vi "Matlab Script.vi"(0 "Xr":dbl[](array[numeric]), 1 "Yr":dbl[](array[numeric]), 2 "Xy":dbl[](array[numeric]), 3 "Yy":dbl[](array[numeric]), 4 "Xw":dbl[](array[numeric]), 5 "Yw":dbl[](array[numeric]), 6 "Couleur Win":u32, 7 "Error In":errorcluster, 10 "Couleur Lose":u32, 11 "Path":path) -> (13 "Error Out":errorcluster, 16 "Script Path 2":path)   [LabVIEW 2025]
doc: "Ce VI construit le script Matlab d’analyse (AnalyseTx.m) à partir des données extraites précédemment\n(Pos.txt) et des paramètres de configuration LabVIEW. Il génère un fichier texte contenant les instructions Matlab prêtes à exécution, en intégrant automatiquement les paramètres. Le fichier Matlab est ensuite enregistré dans le répertoire de travail et sera exécuté par RunMatlab.vi."
panel:
  out "concatenated string":string
  in  "BallminScore":dbl=15.0
  in  "MoveDistPx":dbl=9.0
  in  "BallBorderDist":dbl=9.0
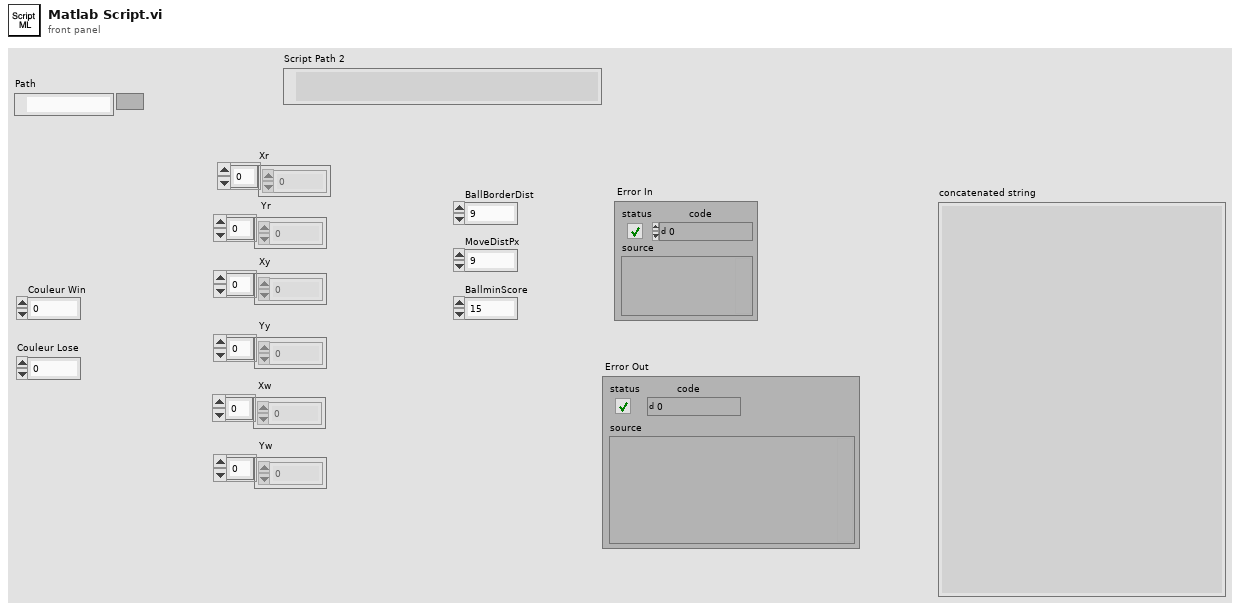
[diagram p1: front panel]
types:
  T1 = enum16{"open", "replace", "create", "open or create", "replace or create", "replace or create with confirmation"}
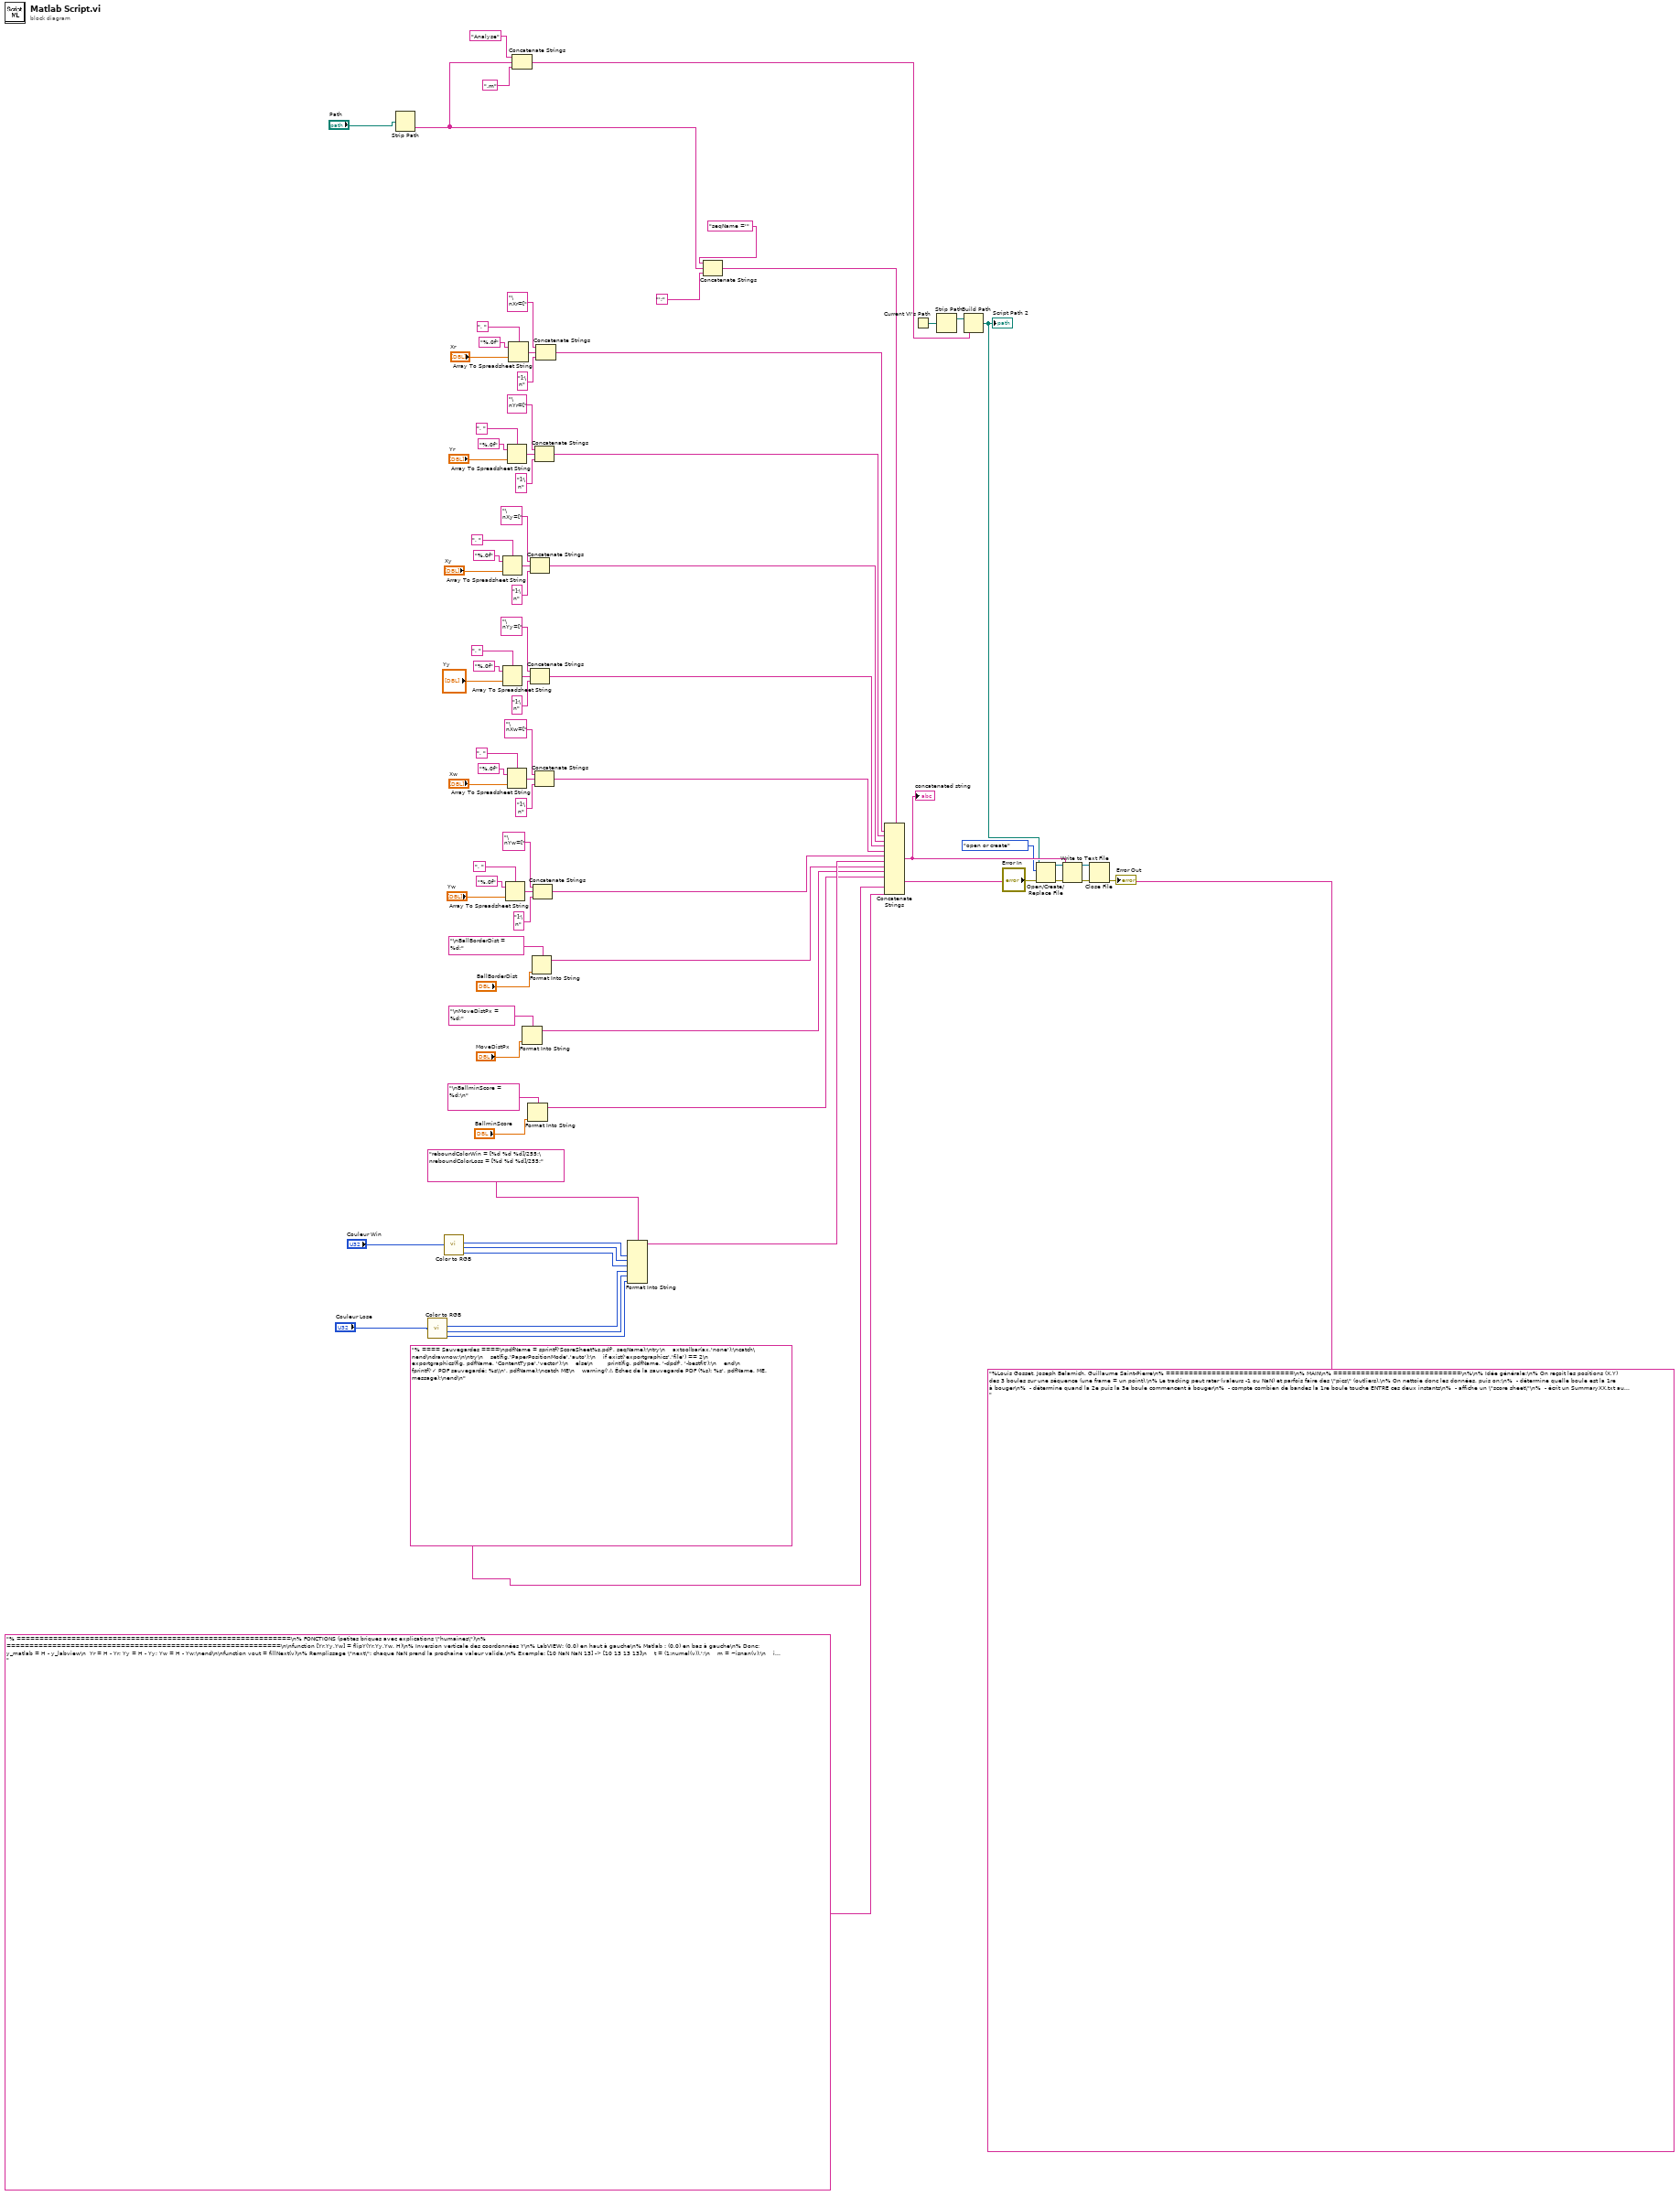
[diagram p0: block diagram]
diagram:
  n1 = Strip Path(path="Path") -> (name=w2:string)  [unwired: 1 out]
  n2 = call <vilib>:"Color to RGB.vi"("Color"="Couleur Lose") -> ("R"=w5:u8, "G"=w4:u8, "B"=w3:u8)  [unwired: 1 out]
  n3 = call <vilib>:"Color to RGB.vi"("Color"="Couleur Win") -> ("R"=w8:u8, "G"=w7:u8, "B"=w6:u8)  [unwired: 1 out]
  n4 = Array To Spreadsheet String(delimiter (Tab)=", ", array="Xy", 3:"%.0f" ("format string")) -> (spreadsheet string=w71:string)
  n5 = Array To Spreadsheet String(delimiter (Tab)=", ", array="Yy", 3:"%.0f" ("format string")) -> (spreadsheet string=w66:string)
  n6 = Array To Spreadsheet String(delimiter (Tab)=", ", array="Yw", 3:"%.0f" ("format string")) -> (spreadsheet string=w56:string)
  n7 = Array To Spreadsheet String(delimiter (Tab)=", ", array="Yr", 3:"%.0f" ("format string")) -> (spreadsheet string=w76:string)
  n8 = Array To Spreadsheet String(delimiter (Tab)=", ", array="Xw", 3:"%.0f" ("format string")) -> (spreadsheet string=w61:string)
  n9 = Array To Spreadsheet String(delimiter (Tab)=", ", array="Xr", 3:"%.0f" ("format string")) -> (spreadsheet string=w81:string)
  n10 = Concatenate Strings("Analyse" ("string"), w2, ".m" ("string")) -> (w40:string)
  n11 = Format Into String(format string="\nMoveDistPx = %d;", "MoveDistPx") -> (resulting string=w10:string)  [unwired: 2 in, 1 out]
  n12 = Format Into String(format string="\nBallminScore = %d;\n", "BallminScore") -> (resulting string=w11:string)  [unwired: 2 in, 1 out]
  n13 = Concatenate Strings("\nXy=[" ("string"), w71, "];\n" ("string")) -> (w37:string)
  n14 = Concatenate Strings("\nYy=[" ("string"), w66, "];\n" ("string")) -> (w36:string)
  n15 = Format Into String(format string="\nBallBorderDist = %d;", "BallBorderDist") -> (resulting string=w12:string)  [unwired: 2 in, 1 out]
  n16 = Concatenate Strings("\nYw=[" ("string"), w56, "];\n" ("string")) -> (w34:string)
  n17 = Concatenate Strings("\nYr=[" ("string"), w76, "];\n" ("string")) -> (w38:string)
  n18 = Concatenate Strings("\nXw=[" ("string"), w61, "];\n" ("string")) -> (w35:string)
  n19 = Concatenate Strings("\nXr=[" ("string"), w81, "];\n" ("string")) -> (w39:string)
  n20 = Format Into String(format string="reboundColorWin = [%d %d %d]/255;\nreboundColorLoss = [%d %d %d]/255;", w8, w7, w6, w5, w4, w3) -> (resulting string=w13:string)  [unwired: 2 in, 1 out]
  n21 = Concatenate Strings("seqName ='" ("string"), w2, "';" ("string")) -> (w19:string)
  n22 = Concatenate Strings(w19, w39, w38, w37, w36, w35, w34, w13, w12, w10, w11, "%Louis Gosset, Joseph Belamich, Guillaume Saint-Pierre\n% ============================\n% MAIN\n% ============================\n%\n% Idée générale:\n% On reçoit les positions (X,Y) des 3 boules sur une séquence (une frame = un point).\n% Le tracking peut rater (valeurs -1 ou NaN) et parfois faire des \"pics\" (outliers).\n% On nettoie donc les données, puis on:\n%  - détermine quelle boule est la 1re à bouger\n%  - détermine quand la 2e puis la 3e boule commencent à bouger\n%  - compte combien de bandes la 1re boule touche ENTRE ces deux instants\n%  - affiche un \"score sheet\"\n%  - écrit un SummaryXX.txt au format imposé (très important pour l'évaluation)\n%\n% Hypothèses de projet:\n% - Si une boule n'est pas trouvée: -1 (ou NaN) => boule \"cachée\", on suppose immobile\n% - Pas de boucle for/while \"inutile\" dans la logique globale (on vectorise autant que possible)\n\n% Les variables suivantes doivent exister avant d'exécuter ce script :\n% seqName, Xr, Yr, Xy, Yy, Xw, Yw, reboundColorWin, reboundColorLoss,\n% BallBorderDist, MoveDistPx, BallminScore\n\n% ------------------------------------------------------------\n% 1) Vérifications d'entrée (on préfère planter tôt avec un message clair)\n% ------------------------------------------------------------\nassertVectorSameLength(Xr, Yr, 'Xr', 'Yr');\nassertVectorSameLength(Xy, Yy, 'Xy', 'Yy');\nassertVectorSameLength(Xw, Yw, 'Xw', 'Yw');\n\n% Option stricte : toutes les séries doivent avoir la même longueur (même nombre de frames)\nL = [numel(Xr), numel(Xy), numel(Xw)];\nif numel(unique(L)) ~= 1\n    error('Analyse:LengthMismatchAll', ...\n        'Toutes les séries doivent avoir la même longueur. Longueurs = [%s].', num2str(L));\nend\n\n% Couleurs utilisées pour dessiner les rebonds selon le verdict (Win/Loss)\nreboundColorWin  = validateMatlabColor(reboundColorWin,  'reboundColorWin');\nreboundColorLoss = validateMatlabColor(reboundColorLoss, 'reboundColorLoss');\n\n% ------------------------------------------------------------\n% 2) Conversion \"valeurs manquantes\" -> NaN\n% ------------------------------------------------------------\n% Dans la partie C / LabVIEW, une boule non trouvée sort souvent en -1,-1.\n% Ici on transforme ça en NaN pour pouvoir traiter proprement ensuite.\nXr(Xr==-1)=NaN;  Xy(Xy==-1)=NaN;  Xw(Xw==-1)=NaN;\nYr(Yr==-1)=NaN;  Yy(Yy==-1)=NaN;  Yw(Yw==-1)=NaN;\n\n% ------------------------------------------------------------\n% 3) Changement de repère: LabVIEW (0,0 en haut-gauche) -> Matlab (0,0 en bas-gauche)\n% ------------------------------------------------------------\nH = 480;                     % hauteur image en pixels (donnée du projet)\n[Yr, Yy, Yw] = flipY(Yr, Yy, Yw, H);\n\n% ------------------------------------------------------------\n% 4) Nettoyage des trajectoires\n% ------------------------------------------------------------\n% Étape A: combler les trous (NaN) par la PROCHAINE valeur valide.\n% Interprétation: \"si elle est cachée quelques frames, on suppose qu'elle n'a pas bougé\".\n[Xr, Yr] = InterpolateNan(Xr, Yr);\n[Xy, Yy] = InterpolateNan(Xy, Yy);\n[Xw, Yw] = InterpolateNan(Xw, Yw);\n\n% Étape B: enlever les \"pics\" de tracking (outliers).\n% Règle: un vrai outlier doit être détecté en X ET en Y, sinon on évite de corriger trop agressivement.\n% Correction: on remplace par la valeur précédente (ça \"recolle\" la trajectoire).\n[Xr, Yr] = RemoveOutlier(Xr, Yr);\n[Xy, Yy] = RemoveOutlier(Xy, Yy);\n[Xw, Yw] = RemoveOutlier(Xw, Yw);\n\n% Étape C: distances parcourues (info affichée dans le PDF)\ndR = GetBallPathLength(Xr, Yr);\ndY = GetBallPathLength(Xy, Yy);\ndW = GetBallPathLength(Xw, Yw);\n\n% ------------------------------------------------------------\n% 5) Déduire le \"cadre\" (les limites du billard) depuis les traces\n% ------------------------------------------------------------\n% Ici on prend simplement min/max de toutes les positions mesurées.\n[Xmin, Xmax, Ymin, Ymax] = GetFrame(Xr, Yr, Xy, Yy, Xw, Yw);\n\n% ------------------------------------------------------------\n% 6) Trouver l'ordre des boules: qui commence à bouger en premier ?\n% ------------------------------------------------------------\n% On dit qu'une boule \"a bougé\" dès qu'elle s'éloigne de son point initial de > MoveDistPx.\niR = GetFirstMoveIdx(Xr, Yr, MoveDistPx);\niY = GetFirstMoveIdx(Xy, Yy, MoveDistPx);\niW = GetFirstMoveIdx(Xw, Yw, MoveDistPx);\n\n% On met Inf si une boule ne bouge jamais (plus simple à trier)\nidx = [inf inf inf];\nif ~isempty(iR), idx(1)=iR; end\nif ~isempty(iY), idx(2)=iY; end\nif ~isempty(iW), idx(3)=iW; end\n\n% Tie-break \"humain\": si 2 boules démarrent au même index, on prend celle\n% dont le tout premier segment est le plus long (ça évite de choisir une boule\n% qui bouge à peine à cause du bruit).\nseg1 = [seglen1(Xr,Yr), seglen1(Xy,Yy), seglen1(Xw,Yw)];\nmins = find(idx == min(idx));\n[~, pick] = max(seg1(mins));\nfirstBall = mins(pick);    % 1=R, 2=Y, 3=W\n\n% On récupère directement la série (X,Y) de la 1re boule\nswitch firstBall\n  case 1, X = Xr; Y = Yr; firstName = 'red';\n  case 2, X = Xy; Y = Yy; firstName = 'yellow';\n  case 3, X = Xw; Y = Yw; firstName = 'white';\nend\ncolorNames    = {'red','yellow','white'};\nfirstBallName = colorNames{firstBall};\n\n% Indices de début de mouvement (Inf si jamais bougé)\nfm = [inf inf inf];\nif ~isempty(iR), fm(1)=iR; end\nif ~isempty(iY), fm(2)=iY; end\nif ~isempty(iW), fm(3)=iW; end\niMoveFirst = fm(firstBall); \n\n% ------------------------------------------------------------\n% 7) Déterminer \"2e boule\" et \"3e boule\" via l'ordre de début de mouvement\n% ------------------------------------------------------------\n[iSecond, iThird, secondBall, thirdBall] = SecondThirdByMove(fm, firstBall); \n\n% ------------------------------------------------------------\n% 8) Détection des rebonds (touches de bandes) pour la 1re boule\n% ------------------------------------------------------------\n% iTouch = indices où on considère qu'il y a \"rebond\".\n% La logique est expliquée dans GetTouchIdx():\n%   - on repère les instants où la boule est proche d'une bande\n%   - et on cherche un changement de signe de vitesse \"normale\" (rebond réel)\n%   - fallback: si pas de changement de signe (rebond glissé), on prend le début\n%     d'une grappe de points proches du bord\n%   - petit anti-bruit (\"debounce\") pour éviter de compter 3 fois le même rebond\niTouch = GetTouchIdx(X, Y, Xmin, Xmax, Ymin, Ymax, BallBorderDist);\n\n% ------------------------------------------------------------\n% 9) Compter les bandes touchées ENTRE la 2e et la 3e boule (début mouvement)\n% ------------------------------------------------------------\nnbBandsBetween = 0;\nif isfinite(iSecond) && isfinite(iThird) && iThird > iSecond\n    nbBandsBetween = nnz( (iTouch >= iSecond) & (iTouch < iThird) );\nend\n\n% Verdict du point: gagné si >=3 bandes entre ces deux instants\nif isfinite(iSecond) && isfinite(iThird) && (nbBandsBetween >= 3)\n    VD = \"Win\";\nelse\n    VD = \"Loss\";\nend\n\n% Couleur d'affichage des rebonds selon Win/Loss\nisWin = strcmpi(char(VD), 'Win');\nif isWin\n    reboundColor = reboundColorWin;\nelse\n    reboundColor = reboundColorLoss;\nend\n\n% Combien de boules ont bougé (utile dans le cartouche)\nnbBallsMoved = sum(isfinite([iR iY iW]));\n\n% ------------------------------------------------------------\n% 10) Affichage \"Scores sheet\"\n% ------------------------------------------------------------\nfig = figure('Color','w','Visible','on'); hold on;\nax = gca; set(ax,'Color','w'); grid(ax,'off'); box(ax,'off');\nax.XTick = []; ax.YTick = []; ax.XMinorTick='off'; ax.YMinorTick='off';\n\n% On ajoute un peu de marge pour pouvoir écrire du texte \"sous\" le billard\npad = 10; padB = 60;\naxis([Xmin-pad, Xmax+pad, Ymin-padB, Ymax+pad]); axis equal; axis off;\n\n% Cadre du billard\nrectangle('Position',[Xmin Ymin (Xmax-Xmin) (Ymax-Ymin)], ...\n          'EdgeColor','b','LineWidth',1);\n\n% Traces (couleurs fixes pour lisibilité)\nplot(Xr, Yr, 'r.-', 'LineWidth',1, 'MarkerSize',6, 'DisplayName','Red');\nplot(Xy, Yy, 'y.-', 'LineWidth',1, 'MarkerSize',6, 'DisplayName','Yellow');\nplot(Xw, Yw, 'b.-', 'LineWidth',1, 'MarkerSize',6, 'DisplayName','White');\n\n% Point initial de chaque boule (étoile/hexagone) -> UNIQUEMENT si la boule a bougé\nmovedR = ~isempty(iR);\nmovedY = ~isempty(iY);\nmovedW = ~isempty(iW);\n\nif movedR && isfinite(Xr(1)) && isfinite(Yr(1))\n    plot(Xr(1), Yr(1), 'rh', 'MarkerSize',20, 'LineWidth',1.2, 'MarkerFaceColor','none');\nend\n\nif movedY && isfinite(Xy(1)) && isfinite(Yy(1))\n    plot(Xy(1), Yy(1), 'yh', 'MarkerSize',20, 'LineWidth',1.2, 'MarkerFaceColor','none', ...\n         'MarkerEdgeColor',[0.85 0.75 0]);\nend\n\nif movedW && isfinite(Xw(1)) && isfinite(Yw(1))\n    plot(Xw(1), Yw(1), 'bh', 'MarkerSize',20, 'LineWidth',1.2, 'MarkerFaceColor','none');\nend\n\n\n% Rebonds UNIQUEMENT entre \"2e bouge\" et \"3e bouge\" (c'est ça qui décide Win/Loss)\niBetween = [];\nif isfinite(iSecond) && isfinite(iThird) && iThird > iSecond && ~isempty(iTouch)\n    iBetween = iTouch( (iTouch >= iSecond) & (iTouch < iThird) );\nend\nif ~isempty(iBetween)\n    hReb = plot(X(iBetween), Y(iBetween), 'o', ...\n        'MarkerSize', 20, 'LineWidth', 1.5, ...\n        'MarkerFaceColor', 'none', ...\n        'DisplayName', 'Rebound 2→3');\n    set(hReb, 'Color', reboundColor, 'MarkerEdgeColor', reboundColor);\nend\n\n% Titre avec timestamp (pratique quand tu génères plusieurs PDF)\nts = datetime('now','Format','dd.MM.yyyy - HH:mm:ss');\ntitle(sprintf('Scores sheet – %s – (%s)', seqName, string(ts)));\n\n% Cartouche texte en bas\nlineGap = 14;  y1 = Ymin - 8;  y2 = y1 - lineGap;  yDist = y1 - 2*lineGap - 2;\ntxtLeft = sprintf('Score sheet for \"%s\"\\n--- %s ---', firstBallName, VD);\ntext(Xmin, y1, txtLeft, 'HorizontalAlignment','left','VerticalAlignment','top', ...\n     'FontName','Helvetica','FontSize',10, 'Color','k', 'Clipping','off');\n\ntext(Xmax, y1, sprintf('%d ball(s) moved', nbBallsMoved), ...\n     'HorizontalAlignment','right','VerticalAlignment','top', ...\n     'FontName','Helvetica','FontSize',10, 'Color','k', 'Clipping','off');\n\ntext(Xmax, y2, sprintf('%d band(s) between 2nd->3rd move', nbBandsBetween), ...\n     'HorizontalAlignment','right','VerticalAlignment','top', ...\n     'FontName','Helvetica','FontSize',10, 'Color','k', 'Clipping','off');\n\ntext(Xmin,            yDist, sprintf('red_{d} : %0.0fpx',   dR), ...\n     'HorizontalAlignment','left','VerticalAlignment','top', ...\n     'FontName','Helvetica','FontSize',10, 'Color','k', 'Clipping','off');\ntext((Xmin+Xmax)/2.0, yDist, sprintf('yellow_{d} : %0.0fpx', dY), ...\n     'HorizontalAlignment','center','VerticalAlignment','top', ...\n     'FontName','Helvetica','FontSize',10, 'Color','k', 'Clipping','off');\ntext(Xmax,            yDist, sprintf('white_{d} : %0.0fpx', dW), ...\n     'HorizontalAlignment','right','VerticalAlignment','top', ...\n     'FontName','Helvetica','FontSize',10, 'Color','k', 'Clipping','off');\n\n% ============================\n% Résumé texte (format imposé)\n% ============================\n% IMPORTANT: ce fichier est parsé automatiquement par l'outil d'évaluation.\n% Donc on respecte STRICTEMENT le format:\n%   f:x; s:x; n:d; b:d; rb:d; yb:d; wb:d;\ntxtName = sprintf('Summary%s.txt', seqName);\nfid = fopen(txtName,'w');\nif fid < 0\n    warning('⚠️ Impossible d''ouvrir %s en écriture.', txtName);\nelse\n    % f : 1re boule (r,y,w)\n    fLetters = {'r','y','w'};\n    fChar = fLetters{firstBall};\n\n    % s : score (w = win, l = loss)\n    if strcmpi(char(VD), 'Win')\n        sChar = 'w';\n    else\n        sChar = 'l';\n    end\n\n    % n : nb de boules ayant bougé\n    nVal = nbBallsMoved;\n\n    % b : nb de bords touchés par la 1re boule (TOUS les rebonds détectés)\n    % (même ceux hors fenêtre 2→3) -> c'est ce qui est demandé dans le summary.\n    bVal = numel(iTouch);\n\n    % rb/yb/wb : distances parcourues (arrondies à l'entier)\n    rbVal = round(dR);\n    ybVal = round(dY);\n    wbVal = round(dW);\n\n    % Ligne EXACTE attendue\n    line = sprintf('f:%s; s:%s; n:%d; b:%d; rb:%d; yb:%d; wb:%d;', ...\n                   fChar, sChar, nVal, bVal, rbVal, ybVal, wbVal);\n\n    fprintf(fid, '%s\\n', line);\n    fclose(fid);\n    fprintf('✓ Résumé sauvegardé: %s\\n', txtName);\nend% ==== Sauvegardes ====\npdfName = sprintf('ScoreSheet%s.pdf', seqName);\ntry\n    axtoolbar(ax,'none');\ncatch\nend\ndrawnow;\n\ntry\n    set(fig,'PaperPositionMode','auto');\n    if exist('exportgraphics','file') == 2\n        exportgraphics(fig, pdfName, 'ContentType','vector');\n    else\n        print(fig, pdfName, '-dpdf', '-bestfit');\n    end\n    fprintf('✓ PDF sauvegardé: %s\\n', pdfName);\ncatch ME\n    warning('⚠️ Échec de la sauvegarde PDF (%s): %s', pdfName, ME.message);\nend", "% ==== Sauvegardes ====\npdfName = sprintf('ScoreSheet%s.pdf', seqName);\ntry\n    axtoolbar(ax,'none');\ncatch\nend\ndrawnow;\n\ntry\n    set(fig,'PaperPositionMode','auto');\n    if exist('exportgraphics','file') == 2\n        exportgraphics(fig, pdfName, 'ContentType','vector');\n    else\n        print(fig, pdfName, '-dpdf', '-bestfit');\n    end\n    fprintf('✓ PDF sauvegardé: %s\\n', pdfName);\ncatch ME\n    warning('⚠️ Échec de la sauvegarde PDF (%s): %s', pdfName, ME.message);\nend\n", "% ============================================================\n% FONCTIONS (petites briques avec explications \"humaines\")\n% ============================================================\n\nfunction [Yr,Yy,Yw] = flipY(Yr,Yy,Yw, H)\n% Inversion verticale des coordonnées Y\n% LabVIEW: (0,0) en haut à gauche\n% Matlab : (0,0) en bas à gauche\n% Donc: y_matlab = H - y_labview\n  Yr = H - Yr; Yy = H - Yy; Yw = H - Yw;\nend\n\nfunction vout = fillNext(v)\n% Remplissage \"next\": chaque NaN prend la prochaine valeur valide.\n% Exemple: [10 NaN NaN 13] -> [10 13 13 13]\n    t = (1:numel(v)).';\n    m = ~isnan(v);\n    if ~any(m), vout = v; return, end\n    vout = interp1(t(m), v(m), t, 'next', 'extrap');\nend\n\nfunction [X, Y] = InterpolateNan(X, Y)\n% Remplit les NaN en X et Y avec la prochaine valeur valide (hypothèse: boule immobile si cachée)\n    sx = size(X); sy = size(Y);\n    X = X(:); Y = Y(:);\n    X = fillNext(X);\n    Y = fillNext(Y);\n    X = reshape(X, sx);\n    Y = reshape(Y, sy);\nend\n\nfunction [X, Y] = RemoveOutlier(X, Y)\n% Enlève les outliers (pics) détectés simultanément en X et Y.\n% Pourquoi X ET Y ?\n% -> sinon un bruit sur une seule coordonnée risquerait de corriger à tort.\n% Remplacement: valeur précédente (solution simple et robuste).\n    sx = size(X); sy = size(Y);\n    Xv = X(:);    Yv = Y(:);\n\n    mX = isoutlier(Xv, 'movmedian', 10);\n    mY = isoutlier(Yv, 'movmedian', 10);\n\n    mask = find(mX & mY);      % indices où X ET Y sont outliers\n    mask(mask == 1) = [];      % évite i-1 invalide\n\n    if isempty(mask)\n        X = reshape(Xv, sx);\n        Y = reshape(Yv, sy);\n        return;\n    end\n\n    mask = sort(mask);\n    for k = 1:numel(mask)\n        i = mask(k);\n        Xv(i) = Xv(i-1);\n        Yv(i) = Yv(i-1);\n    end\n\n    X = reshape(Xv, sx);\n    Y = reshape(Yv, sy);\nend\n\nfunction PathLength = GetBallPathLength(X, Y)\n% Distance totale parcourue = somme des distances entre points successifs\n    X = X(:); Y = Y(:);\n    if numel(X) < 2 || numel(Y) < 2, PathLength = 0; return, end\n    dx = diff(X); dy = diff(Y);\n    PathLength = sum(hypot(dx, dy));\nend\n\nfunction [Xmin, Xmax, Ymin, Ymax] = GetFrame(Xr, Yr, Xy, Yy, Xw, Yw)\n% Cadre minimal englobant toutes les traces (min/max sur toutes les boules)\n    Xall = [Xr(:); Xy(:); Xw(:)];\n    Yall = [Yr(:); Yy(:); Yw(:)];\n    Xmin = min(Xall); Xmax = max(Xall);\n    Ymin = min(Yall); Ymax = max(Yall);\nend\n\nfunction [FirstMoveIdx, MoveDist] = GetFirstMoveIdx(X, Y, MoveDistPx)\n% \"Début de mouvement\" = premier index où la boule s'éloigne du point initial\n% d'une distance > MoveDistPx.\n    if nargin < 3 || isempty(MoveDistPx), MoveDistPx = 9; end\n    X = X(:); Y = Y(:);\n    D = hypot(X - X(1), Y - Y(1));\n    FirstMoveIdx = find(D > MoveDistPx, 1, 'first');\n    if nargout >= 2\n        MoveDist = hypot(diff(X), diff(Y)); \n    end\nend\n\nfunction L = seglen1(X, Y)\n% Longueur du 1er segment (sert uniquement pour départager deux départs \"simultanés\")\n    if numel(X) < 2\n        L = 0;\n    else\n        L = hypot(X(2)-X(1), Y(2)-Y(1));\n    end\nend\n\nfunction idx = firstOfRuns(mask)\n% Renvoie l'index du 1er élément de chaque \"grappe\" de true consécutifs.\n% Exemple: [0 1 1 0 1 1 1 0] -> [2 5]\n    mask = mask(:);\n    idx  = find(mask);\n    if isempty(idx), return; end\n    idx  = idx(:);\n    keep = [true; diff(idx) > 1];\n    idx  = idx(keep);\nend\n\nfunction IdxTouch = GetTouchIdx(X, Y, Xmin, Xmax, Ymin, Ymax, BallBorderDist)\n% Détection \"humaine\" d'un rebond sur bande:\n% 1) La boule doit être proche d'une bande (distance <= BallBorderDist).\n% 2) Idéalement, on veut un rebond \"réel\": la vitesse perpendiculaire à la bande\n%    change de signe (ex: va vers la gauche puis repart vers la droite).\n% 3) Parfois le tracking ne donne pas un changement de signe propre (rebond glissé,\n%    bruit, etc.). Dans ce cas, on prend le début de la grappe \"proche du bord\".\n% 4) On applique un petit anti-doublon temporel (debounce) pour éviter de compter\n%    4 rebonds quand la balle \"tremble\" sur le bord.\n%\n% Important pour ton cas \"double rebond même bande\":\n% - Si la balle repart puis revient, il y aura deux changements de signe => 2 rebonds.\n% - Si elle reste collée au bord sans vraie inversion de direction, on ne comptera\n%   qu'un seul événement (début de grappe), ce qui est volontaire.\n\n    if nargin < 7 || isempty(BallBorderDist), BallBorderDist = 9; end\n    X = X(:); Y = Y(:);\n\n    % Distances à chaque bande\n    dL = X - Xmin;     dR = Xmax - X;\n    dB = Y - Ymin;     dT = Ymax - Y;\n\n    nearL = dL <= BallBorderDist;\n    nearR = dR <= BallBorderDist;\n    nearB = dB <= BallBorderDist;\n    nearT = dT <= BallBorderDist;\n\n    % Vitesses entre échantillons\n    dx = diff(X);\n    dy = diff(Y);\n\n    % sign() renvoie 0 si dx=0, et ça casse la détection de changement de signe.\n    % Donc on \"remplace\" les zéros par le signe voisin.\n    sdx = signNoZero(dx);\n    sdy = signNoZero(dy);\n\n    % Changements de signe: indicateurs de rebond \"propre\"\n    turnNegPosX = (sdx(1:end-1) < 0) & (sdx(2:end) > 0);  % allait vers -X puis +X => rebond à gauche\n    turnPosNegX = (sdx(1:end-1) > 0) & (sdx(2:end) < 0);  % rebond à droite\n    turnNegPosY = (sdy(1:end-1) < 0) & (sdy(2:end) > 0);  % rebond en bas\n    turnPosNegY = (sdy(1:end-1) > 0) & (sdy(2:end) < 0);  % rebond en haut\n\n    % +1 pour revenir à l'index \"dans\" X,Y (car turn est calculé sur diff)\n    iL = find(turnNegPosX) + 1;  iL = iL(nearL(iL));\n    iR = find(turnPosNegX) + 1;  iR = iR(nearR(iR));\n    iB = find(turnNegPosY) + 1;  iB = iB(nearB(iB));\n    iT = find(turnPosNegY) + 1;  iT = iT(nearT(iT));\n\n    % Fallback: pas de changement de signe détectable => rebond \"glissé\" ou bruit\n    if isempty(iL), iL = firstOfRuns(nearL); end\n    if isempty(iR), iR = firstOfRuns(nearR); end\n    if isempty(iB), iB = firstOfRuns(nearB); end\n    if isempty(iT), iT = firstOfRuns(nearT); end\n\n    % On ignore l'index 1 (souvent faux positif: position initiale déjà proche du bord)\n    iL(iL==1) = []; iR(iR==1) = []; iB(iB==1) = []; iT(iT==1) = [];\n\n    % Anti-doublons (si bruit): on force un espacement minimal entre événements\n    minGap = 2; % en frames\n    iL = debounceIdx(iL, minGap);\n    iR = debounceIdx(iR, minGap);\n    iB = debounceIdx(iB, minGap);\n    iT = debounceIdx(iT, minGap);\n\n    % Merge des rebonds détectés (unique = si un rebond coin doit compter 2 bandes, enlever unique())\n    IdxTouch = sort(unique([iL; iR; iB; iT]));\nend\n\nfunction s = signNoZero(v)\n% But: éviter les zéros dans sign(v), sinon un vrai rebond peut ne pas être vu.\n% On remplit les 0 avec le signe précédent/suivant.\n    s = sign(v);\n    s(s==0) = NaN;\n    s = fillmissing(s, 'previous');\n    s = fillmissing(s, 'next');\n    s(isnan(s)) = 0;\nend\n\nfunction idx = debounceIdx(idx, gap)\n% Garde uniquement les événements espacés d'au moins \"gap\" frames.\n% Exemple: [10 11 12 30] avec gap=2 -> [10 30]\n    idx = idx(:);\n    if isempty(idx), return; end\n    keep = [true; diff(idx) > gap];\n    idx = idx(keep);\nend\n\nfunction [iSecond, iThird, secondBall, thirdBall] = SecondThirdByMove(firstMoveIdx, firstBall)\n% On veut \"2e\" et \"3e\" boules selon leur début de mouvement (pas selon la couleur).\n% Si une boule ne bouge pas: Inf => on ne peut pas établir 2e/3e correctement.\n    others = setdiff(1:3, firstBall);\n    candIdx  = [firstMoveIdx(others(1)), firstMoveIdx(others(2))];\n    candBall = [others(1),                 others(2)];\n    m = isfinite(candIdx);\n\n    if nnz(m) < 2\n        iSecond = inf; iThird = inf; secondBall = NaN; thirdBall = NaN;\n        return;\n    end\n\n    candIdx  = candIdx(m);\n    candBall = candBall(m);\n    [~,ord]  = sort(candIdx, 'ascend');\n    candIdx  = candIdx(ord);\n    candBall = candBall(ord);\n\n    iSecond    = candIdx(1);\n    iThird     = candIdx(2);\n    secondBall = candBall(1);\n    thirdBall  = candBall(2);\nend\n\nfunction assertVectorSameLength(X, Y, nameX, nameY)\n% Petites vérifs \"anti-galère\":\n% - numériques\n% - vecteurs\n% - pas vides\n% - même taille\n    if ~isnumeric(X) || ~isnumeric(Y)\n        error('Analyse:TypeError', '%s et %s doivent être numériques.', nameX, nameY);\n    end\n    if ~isvector(X) || ~isvector(Y)\n        error('Analyse:NotVector', '%s et %s doivent être des vecteurs.', nameX, nameY);\n    end\n    if isempty(X) || isempty(Y)\n        error('Analyse:EmptyVector', '%s ou %s est vide.', nameX, nameY);\n    end\n    if numel(X) ~= numel(Y)\n        error('Analyse:LengthMismatchPair', ...\n            'Longueur différente: %s=%d, %s=%d.', nameX, numel(X), nameY, numel(Y));\n    end\nend\n\nfunction c = validateMatlabColor(cIn, argName)\n% Accepte:\n%  - 'r','g','b','c','m','y','k','w'\n%  - [r g b] avec r,g,b dans [0..1] (format Matlab)\n%\n% But: éviter de découvrir au milieu du script que la couleur est invalide.\n    if isstring(cIn) && isscalar(cIn), cIn = char(cIn); end\n\n    if ischar(cIn)\n        if numel(cIn) ~= 1 || ~ismember(cIn, ['r','g','b','c','m','y','k','w'])\n            error('Analyse:BadColorChar', ...\n                '%s doit être une lettre parmi r g b c m y k w (ex: ''g'').', argName);\n        end\n        c = cIn;\n        return\n    end\n\n    if isnumeric(cIn) && numel(cIn) == 3\n        c = double(cIn(:)).';\n        if any(~isfinite(c))\n            error('Analyse:BadColorNaNInf', '%s contient NaN/Inf.', argName);\n        end\n        if any(c < 0 | c > 1)\n            error('Analyse:BadColorRGB', ...\n                '%s doit être [r g b] dans [0..1]. Reçu: [%g %g %g].', argName, c(1), c(2), c(3));\n        end\n        return\n    end\n\n    error('Analyse:BadColorType', ...\n        '%s doit être une lettre (''g'') ou un RGB 1x3 dans [0..1].', argName);\nend") -> (w32:string)
  "concatenated string" <- w32
  n23 = Current VI's Path() -> (path=w23:path)
  n24 = Strip Path(path=w23) -> (stripped path=w22:path)  [unwired: 1 out]
  n25 = Build Path(base path=w22, name or relative path=w40) -> (appended path=w31:path)
  "Script Path 2" <- w31
  n26 = Open/Create/Replace File(file path (use dialog)=w31, error in="Error In", operation (0:open)=T1."open or create") -> (refnum out=w30:refnum<file>, error out=w29:errorcluster)  [unwired: 3 in, 1 out]
  n27 = Write to Text File(file (use dialog)=w30, text=w32, error in=w29) -> (refnum out=w27:refnum<file>, error out=w25:errorcluster)  [unwired: 1 in, 1 out]
  n28 = Close File(refnum=w27, error in=w25) -> (error out=→"Error Out":errorcluster)  [unwired: 1 out]
